vi "GetPigeonIMU.vi"(8 "Reset Yaw (deg)":dbl format="%#_13g", 11 "Reset Yaw":bool) -> (1 "Roll (deg)":dbl format="%#_13g", 2 "Pitch (deg)":dbl format="%#_13g", 3 "Yaw (deg)":dbl format="%#_13g")   [LabVIEW 2019]
doc: "This VI reads the Pigeon IMU yaw, pitch, and roll values. It also handles error detection and orientation resets."
uses:
  refnums.vi
  <vilib>/Rock Robotics/WPI/ThirdParty/Phoenix-LabVIEW/Pigeon IMU/CTRE_PigeonIMU_GetYPR.vi
  sensors.vi
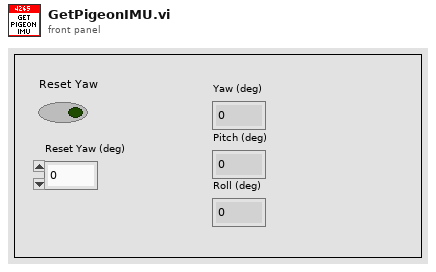
[diagram p1: front panel]
types:
  T1 = typedef "CTRE_PigeonIMU_DeviceRef.ctl" = cluster{"DeviceStatus":errorcluster, "Device Number":u8, "Type":T2, "Device ID":u32, "Handle":u64, "UsageFrame":u32, "Library Path":path}
  T2 = typedef "CTRE_PigeonIMU_ConnectionType.ctl" = u32
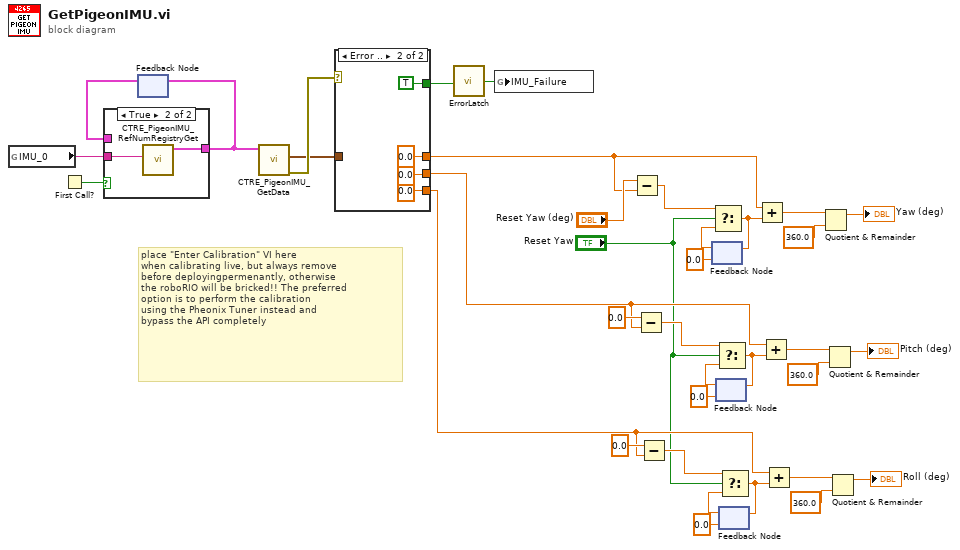
[diagram p0: block diagram]
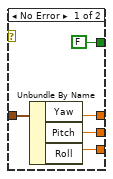
[diagram p2: hidden frame]
diagram:
  # "place \"Enter Calibration\" VI here\nwhen calibrating live, but always remove \nbefore deployingpermenantly, otherwise \nthe roboRIO will be bricked!! The preferred\noption is to perform the calibration\nusing the Pheonix Tuner instead and\nbypass the API completely"
  n1 = global read "refnums.vi" "IMU_0"() -> (w34:string)
  n2 = First Call?() -> (First Call?: T/F=w36:bool)
  n3 = feedback #1() -> (w35:T1)  [unwired: 1 in]
  n4 = case shown="True" w36 {
    tunnel: [w37 w39] -> w33
    tunnel: w35 -> [w37 _]
    tunnel: w34 -> [_ w38]
    frame False {
    }
    frame True {
      n5 = call <vilib>:"CTRE_PigeonIMU_RefNumRegistryGet.vi"("refnum name"=w38) -> ("PigeonIMUDevRef"=w39:T1)  [unwired: 9 in, 1 out]
    }
  }
  n6 = feedback-in #1(w33) -> ()
  n7 = call-poly <vilib>:"CTRE_PigeonIMU_GetData.vi"("PigeonIMUDevRef"=w33) -> ("error out"=w24:errorcluster, "Yaw Pitch Roll"=w21:cluster{"Yaw":dbl, "Pitch":dbl, "Roll":dbl})  [unwired: 8 in, 1 out]
  n8 = case shown="Error .." w24 {
    tunnel: [FALSE TRUE] -> w23
    tunnel: w21 -> [w43 _]
    tunnel: [w42 0.0 ("Yaw")] -> w20
    tunnel: [w41 0.0 ("Pitch")] -> w11
    tunnel: [w40 0.0 ("Roll")] -> w2
    frame No Error {
      n9 = Unbundle By Name(w43) -> ("Yaw"=w42:dbl, "Pitch"=w41:dbl, "Roll"=w40:dbl)
    }
    frame Error {
    }
  }
  n10 = call "ErrorLatch.vi"("Trigger"=w23) -> ("Latched"=w22:bool)
  n11 = global write "sensors.vi" "IMU_Failure"(w22) -> ()
  n12 = Subtract(x="Reset Yaw (deg)", y=w20) -> (x-y=w32:dbl)
  n13 = Subtract(x=0.0, y=w11) -> (x-y=w19:dbl)
  n14 = Subtract(x=0.0, y=w2) -> (x-y=w10:dbl)
  n15 = feedback #2(0.0) -> (w31:dbl)
  n16 = Select(t=w32, s="Reset Yaw", f=w31) -> (s? t:f=w29:dbl)
  n17 = feedback-in #2(w29) -> ()
  n18 = feedback #3(0.0) -> (w18:dbl)
  n19 = Select(t=w19, s="Reset Yaw", f=w18) -> (s? t:f=w16:dbl)
  n20 = feedback-in #3(w16) -> ()
  n21 = feedback #4(0.0) -> (w9:dbl)
  n22 = Select(t=w10, s="Reset Yaw", f=w9) -> (s? t:f=w7:dbl)
  n23 = feedback-in #4(w7) -> ()
  n24 = Add(x=w20, y=w29) -> (x+y=w26:dbl)
  n25 = Add(x=w11, y=w16) -> (x+y=w14:dbl)
  n26 = Add(x=w2, y=w7) -> (x+y=w5:dbl)
  n27 = Quotient & Remainder(x=w26, y=360.0) -> (x-y*floor(x/y)=→"Yaw (deg)":dbl)  [unwired: 1 out]
  n28 = Quotient & Remainder(x=w14, y=360.0) -> (x-y*floor(x/y)=→"Pitch (deg)":dbl)  [unwired: 1 out]
  n29 = Quotient & Remainder(x=w5, y=360.0) -> (x-y*floor(x/y)=→"Roll (deg)":dbl)  [unwired: 1 out]
